vi "CLI_CreateCmdLine.vi"(8 "error in (no error)":errorcluster caption="entrée d'erreur (pas d'erreur)", 10 "ParsedParametersIn":cluster{"Name":string, "Value":string}[](array[cluster]), 11 "CmdLineIn":string) -> (0 "Error out":errorcluster, 3 "CmdLineOut":string)   [LabVIEW 2013]
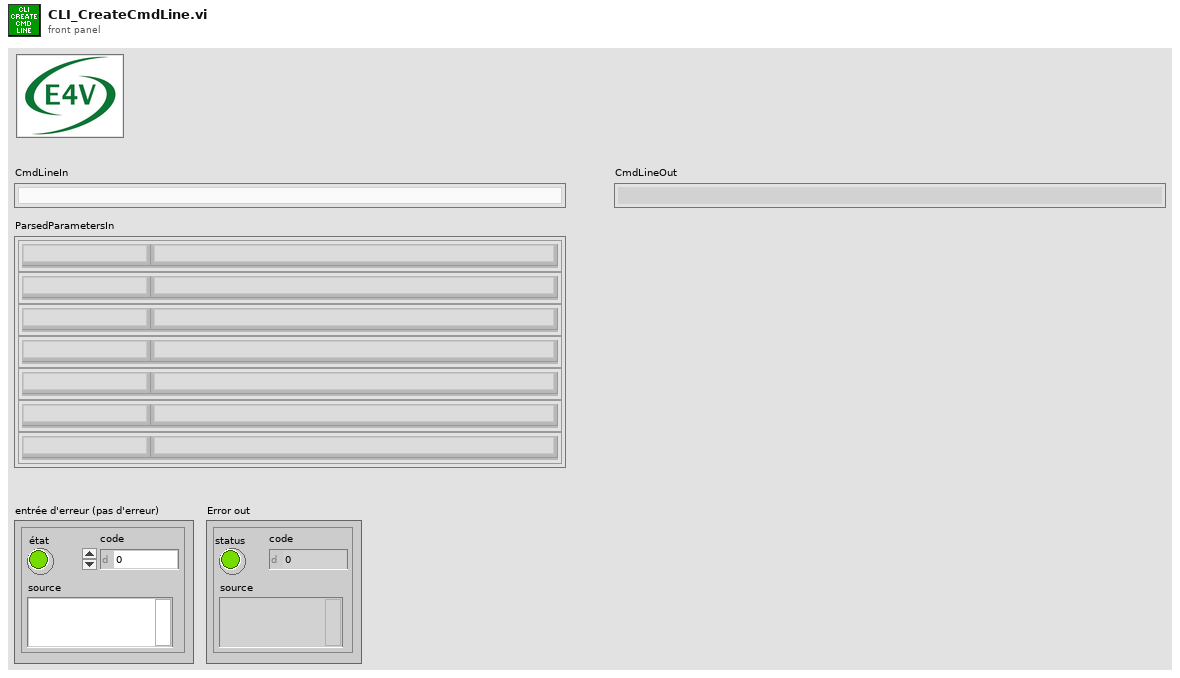
[diagram p1: front panel]
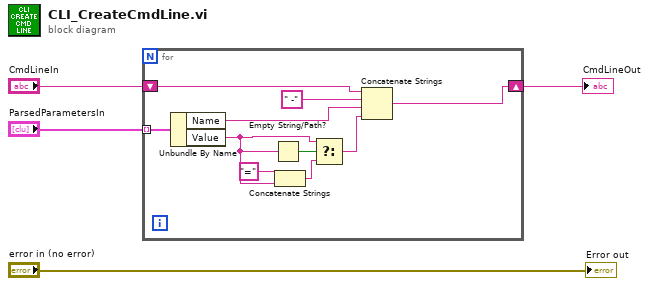
[diagram p0: block diagram]
diagram:
  n1 = for {
    tunnel: "ParsedParametersIn" -> [w14] mode=indexing
    shift-right: [w10] -> w2
    shift-left: "CmdLineIn" -> [w11]
    n2 = Unbundle By Name(w14) -> ("Name"=w12:string, "Value"=w7:string)
    n3 = Empty String/Path?(string/path=w7) -> (empty?=w8:bool)
    n4 = Concatenate Strings("=", w7) -> (w5:string)
    n5 = Select(t=w7, s=w8, f=w5) -> (s? t:f=w6:string)
    n6 = Concatenate Strings(w11, " -", w12, w6) -> (w10:string)
  }
  "CmdLineOut" <- w2
  "Error out" <- "error in (no error)"
